vi "test_Add Single Ch. Enumerated List.vi"(8 "error in (no error)":errorcluster, 11 "TestCase in":refnum<class "Instrument Addon Scripting API Channels Unit Tests.lvclass">) -> (0 "error out":errorcluster, 3 "TestCase out":refnum<class "Instrument Addon Scripting API Channels Unit Tests.lvclass">)   [LabVIEW 2018, in "Instrument Addon Scripting API Channels Unit Tests.lvclass"]
uses:
  Instrument Addon Scripting API Channels Unit Tests.lvclass
  APIs/Scripting API/TypeDefs/Single Channel Enumerated List Settings.ctl
  Addon/Addon Shared/Types/Protocol Data Type.ctl
  Addon/Addon Shared/Types/Data Channel Type.ctl
  Instrument Addon Scripting API Channels Unit Tests.lvclass/Instrument Addon Scripting API Channels Unit Tests.ctl
  Addon/Addon Shared/SubVIs/Constants.vi
  <vilib>/NI/NI VeriStand Advanced SysDef API/_SubVIs/SysDef.Search.GUID.vi
  <vilib>/NI/NI VeriStand Advanced SysDef API/_SubVIs/SysDef.Search.GUIDs.vi
  APIs/Scripting API/Channels/Create Data Channel - Single Channel - Enumerated List.vi
  <vilib>/NI Veristand/Custom Device API/Get Item Property (U16).vi
  <vilib>/NI Veristand/Custom Device API/Get Item Property (String Array).vi
  <vilib>/addons/_JKI Toolkits/VI Tester/TestCase.llb/TestCase.lvclass
  Instrument Addon Scripting API Test Assets/Instrument Addon Scripting API Test Assets.lvclass
  <vilib>/NI/NI VeriStand Advanced SysDef API/SysDef API/Advanced System Definition.lvlib
  Addon/Addon Shared/Instrument Addon Shared.lvlib
  APIs/Scripting API/Instrument Addon Scripting API.lvlib
  <vilib>/NI Veristand/Custom Device API/Custom Device API.lvlib
  C:/Program Files (x86)/National Instruments/LabVIEW 2018/vi.lib/addons/_JKI Toolkits/VI Tester/TestCase.llb/TestCase.lvclass
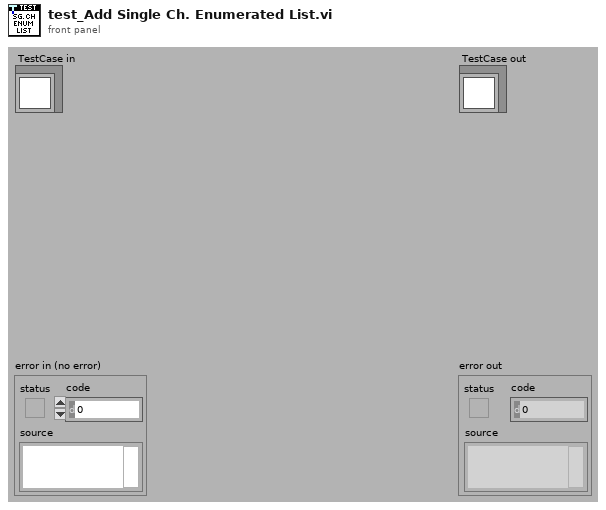
[diagram p1: front panel]
types:
  T1 = typedef "Instrument Addon Scripting API.lvlib/Single Channel Enumerated List Settings.ctl" = cluster{"Enumerated List":string[], "Default Value":dbl, "Units":string}
  T2 = typedef "Instrument Addon Shared.lvlib/Data Channel Type.ctl" = enum16{"Format", "Comparison", "Type Cast", "Enumerated List"}
  T3 = typedef "Instrument Addon Shared.lvlib/Protocol Data Type.ctl" = enum16{"Single Channel", "Array"}
  T4 = typedef "Custom Device API.lvlib/Custom Device Item Ref.ctl" = u64
  T5 = typedef "Custom Device API.lvlib/Custom Device Channel.ctl" = cluster{"Type":T6, "Units":string, "Default Value":dbl, "Faultable":bool, "Scalable":bool}
  T6 = typedef "Custom Device API.lvlib/Custom Device Channel Type.ctl" = enum16{"Input", "Output"}
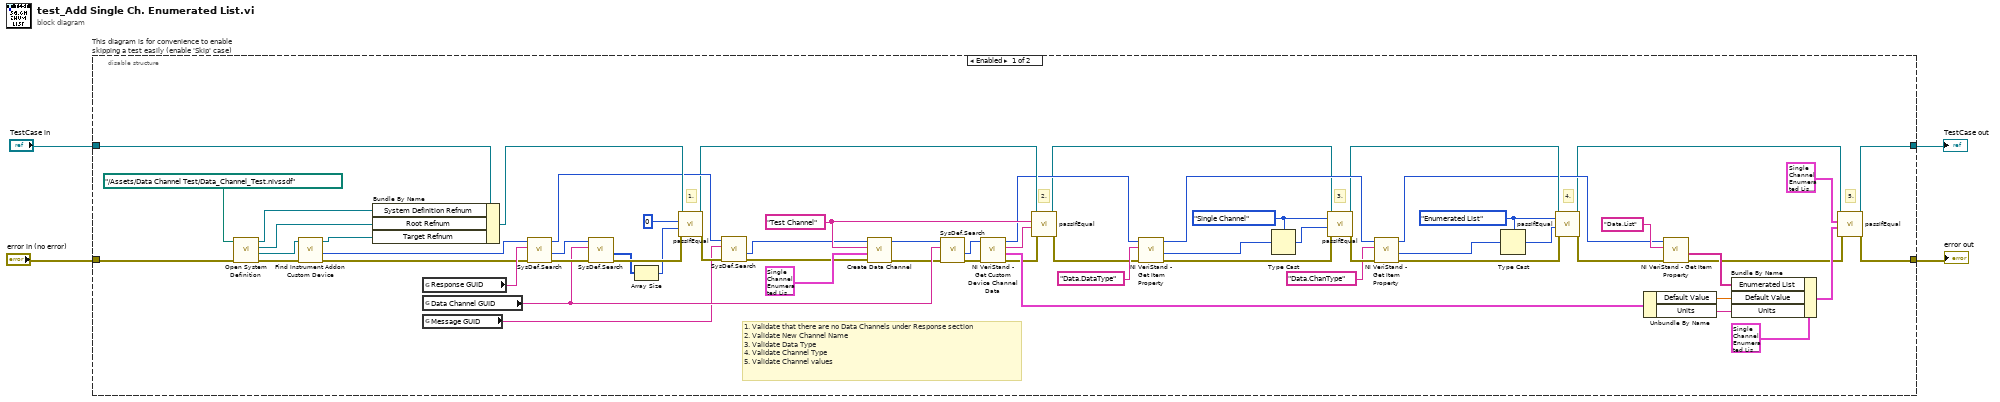
[diagram p0: block diagram]
diagram:
  n1 = disable-structure "This diagram is for convenience to enable skipping a test easily (enable 'Skip' case)" shown="Enabled" {
    disable-tunnel: "TestCase in" -> [w33 w71]
    disable-tunnel: [w67 w69] -> w1
    disable-tunnel: [w66 w70] -> w3
    disable-tunnel: "error in (no error)" -> [w62 w68]
    frame Enabled {
      w16 = Data_Channel_Type."Enumerated List" ("Channel Type")
      w21 = Protocol_Data_Type."Single Channel" ("Data Type")
      w41 = "Test Channel" ("Name")
      # "1. Validate that there are no Data Channels under Response section\n2. Validate New Channel Name\n3. Validate Data Type\n4. Validate Channel Type\n5. Validate Channel values"
      # "4."
      # "3."
      # "5."
      # "2."
      # "1."
      n2 = call "Open System Definition.vi"("error in (no error)"=w62, "System Definition File"=path "../Assets/Data Channel Test/Data_Channel_Test.nivssdf") -> ("error out"=w65:errorcluster, "Target Refnum"=w64:refnum<k24>, "Root Refnum"=w36:refnum<k24>, "System Definition Refnum"=w37:refnum<k24>)  [unwired: 6 in]
      n3 = call "Find Instrument Addon Custom Device.vi"("error in"=w65, "target in"=w64) -> ("error out"=w34:errorcluster, "NodeID"=w61:u64, "target out"=w35:refnum<k24>)  [unwired: 7 in]
      n4 = Bundle By Name(cluster=w33, "System Definition Refnum"=w37, "Root Refnum"=w36, "Target Refnum"=w35) -> (w32:refnum<class "Instrument Addon Scripting API Channels Unit Tests.lvclass">)
      n5 = global read "Constants.vi" "Response GUID"() -> (w60:string)
      n6 = global read "Constants.vi" "Data Channel GUID"() -> (w57:string)
      n7 = global read "Constants.vi" "Message GUID"() -> (w29:string)
      n8 = call-poly <vilib>:"SysDef.Search.vi"("error in (no error)"=w34, "GUID"=w60, "nodeID"=w61) -> ("error out"=w58:errorcluster, "Value out"=w59:u64, "nodeID out"=w28:u64)  [unwired: 5 in, 1 out]
      n9 = call-poly <vilib>:"SysDef.Search.vi"("error in (no error)"=w58, "GUID"=w57, "nodeID"=w59) -> ("error out"=w46:errorcluster, "Values Out"=w45:u64[])  [unwired: 5 in, 2 out]
      n10 = Array Size(array=w45) -> (size(s)=w44:i32)
      n11 = call-dynamic "passIfEqual.vi"("error in (no error)"=w46, "y"=w44, "x"=0 ("size(s)"), "TestCase in"=w32) -> ("error out"=w31:errorcluster, "TestCase out"=w26:refnum<class "Instrument Addon Scripting API Channels Unit Tests.lvclass">)  [unwired: 6 in]
      n12 = call-poly <vilib>:"SysDef.Search.vi"("error in (no error)"=w31, "GUID"=w29, "nodeID"=w28) -> ("error out"=w30:errorcluster, "Value out"=w27:u64)  [unwired: 5 in, 2 out]
      n13 = call-poly "Create Data Channel.vi"("Error In"=w30, "Settings"=T1 {"Enumerated List"=["Test List Element 1"], "Default Value"=10.0, "Units"="ms"}, "Name"=w41, "Message Refnum In"=w27) -> ("Error Out"=w38:errorcluster, "Message Refnum Out"=w39:T4)  [unwired: 5 in, 1 out]
      n14 = call-poly <vilib>:"SysDef.Search.vi"("error in (no error)"=w38, "GUID"=w57, "nodeID"=w39) -> ("error out"=w56:errorcluster, "Value out"=w55:u64)  [unwired: 5 in, 2 out]
      n15 = call <vilib>:"NI VeriStand - Get Custom Device Channel Data.vi"("error in (no error)"=w56, "Channel Ref in"=w55) -> ("error out"=w11:errorcluster, "Channel"=w52:T5, "Channel Name"=w48:string, "Channel Ref out"=w12:T4)  [unwired: 4 in, 2 out]
      n16 = call-dynamic "passIfEqual.vi"("error in (no error)"=w11, "y"=w48, "x"=w41, "TestCase in"=w26) -> ("error out"=w10:errorcluster, "TestCase out"=w9:refnum<class "Instrument Addon Scripting API Channels Unit Tests.lvclass">)  [unwired: 6 in]
      n17 = call-poly <vilib>:"NI VeriStand - Get Item Property.vi"("error in (no error)"=w10, "Property Name"="Data.DataType", "Item Ref in"=w12) -> ("error out"=w24:errorcluster, "Value"=w23:u16, "Item Ref out"=w15:T4)  [unwired: 5 in, 1 out]
      n18 = Type Cast(type=w21, x=w23) -> (*(type *) &x=w22:T3)
      n19 = call-dynamic "passIfEqual.vi"("error in (no error)"=w24, "y"=w22, "x"=w21, "TestCase in"=w9) -> ("error out"=w20:errorcluster, "TestCase out"=w13:refnum<class "Instrument Addon Scripting API Channels Unit Tests.lvclass">)  [unwired: 6 in]
      n20 = call-poly <vilib>:"NI VeriStand - Get Item Property.vi"("error in (no error)"=w20, "Property Name"="Data.ChanType", "Item Ref in"=w15) -> ("error out"=w19:errorcluster, "Value"=w18:u16, "Item Ref out"=w7:T4)  [unwired: 5 in, 1 out]
      n21 = Type Cast(type=w16, x=w18) -> (*(type *) &x=w17:T2)
      n22 = call-dynamic "passIfEqual.vi"("error in (no error)"=w19, "y"=w17, "x"=w16, "TestCase in"=w13) -> ("error out"=w8:errorcluster, "TestCase out"=w6:refnum<class "Instrument Addon Scripting API Channels Unit Tests.lvclass">)  [unwired: 6 in]
      n23 = Unbundle By Name(w52) -> ("Default Value"=w51:dbl, "Units"=w50:string)
      n24 = call-poly <vilib>:"NI VeriStand - Get Item Property.vi"("error in (no error)"=w8, "Property Name"="Data.List", "Item Ref in"=w7) -> ("error out"=w5:errorcluster, "Value"=w53:string[])  [unwired: 5 in, 2 out]
      n25 = Bundle By Name(cluster=T1 {"Enumerated List"=["Test List Element 1"], "Default Value"=10.0, "Units"="ms"} ("Settings"), "Enumerated List"=w53, "Default Value"=w51, "Units"=w50) -> (w47:T1)
      n26 = call-dynamic "passIfEqual.vi"("error in (no error)"=w5, "y"=w47, "x"=T1 {"Enumerated List"=["Test List Element 1"], "Default Value"=10.0, "Units"="ms"} ("Settings"), "TestCase in"=w6) -> ("error out"=w66:errorcluster, "TestCase out"=w67:refnum<class "Instrument Addon Scripting API Channels Unit Tests.lvclass">)  [unwired: 6 in]
    }
    frame Disabled {
      # "skip test result while test is under development"
      n27 = call <vilib>:"skip.vi"("error in (no error)"=w68, "TestCase in"=w71) -> ("error out"=w70:errorcluster, "TestCase out"=w69:refnum<class "Instrument Addon Scripting API Channels Unit Tests.lvclass">)  [unwired: 8 in]
    }
  }
  "error out" <- w3
  "TestCase out" <- w1
